vi "SOMETHING.vi"(4 "User Parameter":variant, 5 "Event Data":cluster{"sender":refnum<k24>, "e":refnum<k24>}, 6 "Control Ref":refnum<k24>, 7 "Event Common Data":T1) -> ()   [LabVIEW 2011]
uses:
  Microsoft.Kinect
  Desktop/Kinect Mouse/Kinect/Kinect Global Status.vi
panel:
  in  "User Parameter 2":variant
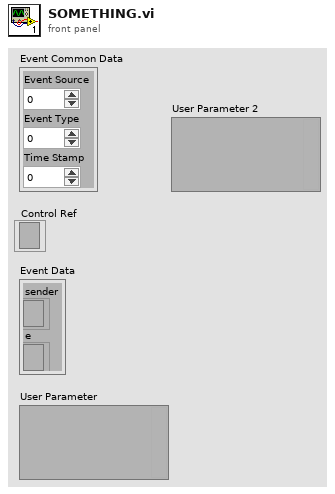
[diagram p1: front panel]
types:
  T1 = cluster{"Event Source":i32, "Event Type":u32, "Time Stamp":u32}
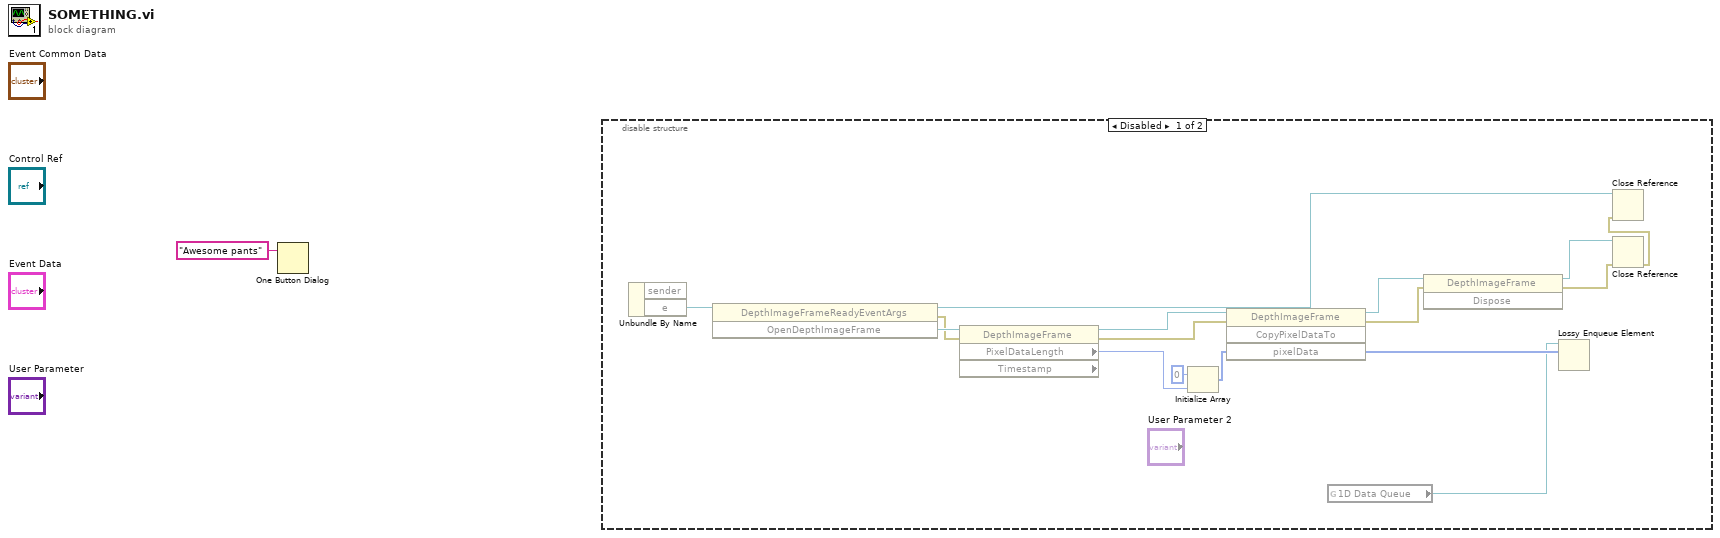
[diagram p0: block diagram]
diagram:
  n1 = One Button Dialog(message="Awesome pants") -> ()  [unwired: 1 in, 1 out]
  n2 = disable-structure shown="Disabled" {
    frame Disabled {
      n3 = Unbundle By Name() -> ("e"=w15:refnum<k24>)  [unwired: 1 in, 1 out]
      n4 = invoke class="DepthImageFrameReadyEventArgs" method="OpenDepthImageFrame"(reference=w15) -> (reference out=w13:refnum<k24>, error out=w16:errorcluster, "OpenDepthImageFrame"=w17:refnum<k24>)  [unwired: 2 in]
      n5 = property on="Property Node" class="DepthImageFrame" props=["PixelDataLength", "Timestamp"](reference=w17, error in=w16) -> (reference out=w8:refnum<k24>, error out=w10:errorcluster, "PixelDataLength"=w3:i32)  [unwired: 1 out]
      n6 = Initialize Array(i16 0 ("element"), w3) -> (w4:i16[])
      n7 = invoke class="DepthImageFrame" method="CopyPixelDataTo"(reference=w8, error in=w10, "pixelData"=w4) -> (reference out=w7:refnum<k24>, error out=w9:errorcluster, "pixelData"=w6:i16[])  [unwired: 1 in, 1 out]
      n8 = global read "Kinect Global Status.vi" "1D Data Queue"() -> (w2:refnum<queue>)
      n9 = invoke class="DepthImageFrame" method="Dispose"(reference=w7, error in=w9) -> (reference out=w14:refnum<k24>, error out=w12:errorcluster)  [unwired: 1 in, 1 out]
      n10 = Lossy Enqueue Element(queue=w2, element=w6) -> ()  [unwired: 1 in, 4 out]
      n11 = Close Reference(reference=w14, error in (no error)=w12) -> (error out=w11:errorcluster)
      n12 = Close Reference(reference=w13, error in (no error)=w11) -> ()  [unwired: 1 out]
    }
    frame Enabled {
    }
  }
